vi "AB_1200_1100_Project_Source_ExportedAssemblyVI.vi"(7 "action":T4, 8 "error in (no error)":errorcluster, 9 "index in":i32, 10 "dataSource in":cluster{"ExportAssemblyVIinfo":T2}, 11 "buildObject":T1) -> (0 "error out":errorcluster, 1 "index out":i32, 2 "dataSource out":cluster{"ExportAssemblyVIinfo":T2}, 3 "buildObject out":T1)   [LabVIEW 2020]
doc: "Reads and writes the data to the object property bag."
uses:
  <vilib>/AppBuilder/RW_Project/AB_RW_Project_PropBag_Action.ctl
  <vilib>/AppBuilder/AB_InteropAssembly_DistVI_Proto_Info.ctl
  <vilib>/AppBuilder/IOStatus.ctl
  <resource>/Framework/Providers/API/ItemRef.ctl
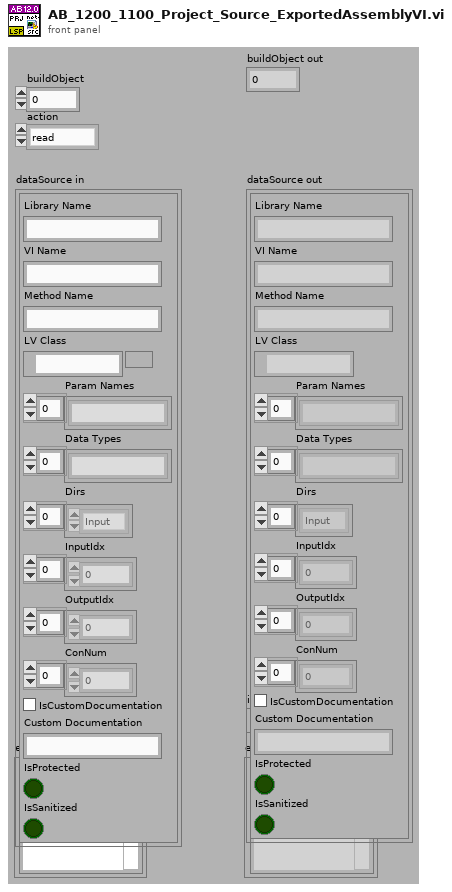
[diagram p1: front panel]
types:
  T1 = typedef "ItemRef.ctl" = u64
  T2 = typedef "AB_InteropAssembly_DistVI_Proto_Info.ctl" = cluster{"Library Name":string, "VI Name":string, "Method Name":string, "LV Class":path, "Param Names":string[], "Data Types":string[], "Dirs":T3[], "InputIdx":i32[], "OutputIdx":i32[], "ConNum":i8[], "IsCustomDocumentation":bool, "Custom Documentation":string, "IsProtected":bool, "IsSanitized":bool}
  T3 = typedef "IOStatus.ctl" = enum16{"Input", "Output", "Input/Output", "InputDeleted", "OutputDeleted", "IODeleted", "ErrorClusterIn", "ErrorClusterOut"}
  T4 = typedef "AB_RW_Project_PropBag_Action.ctl" = enum16{"read", "write", "clear", "readPrevious", "writePrevious", "clearPrevious"}
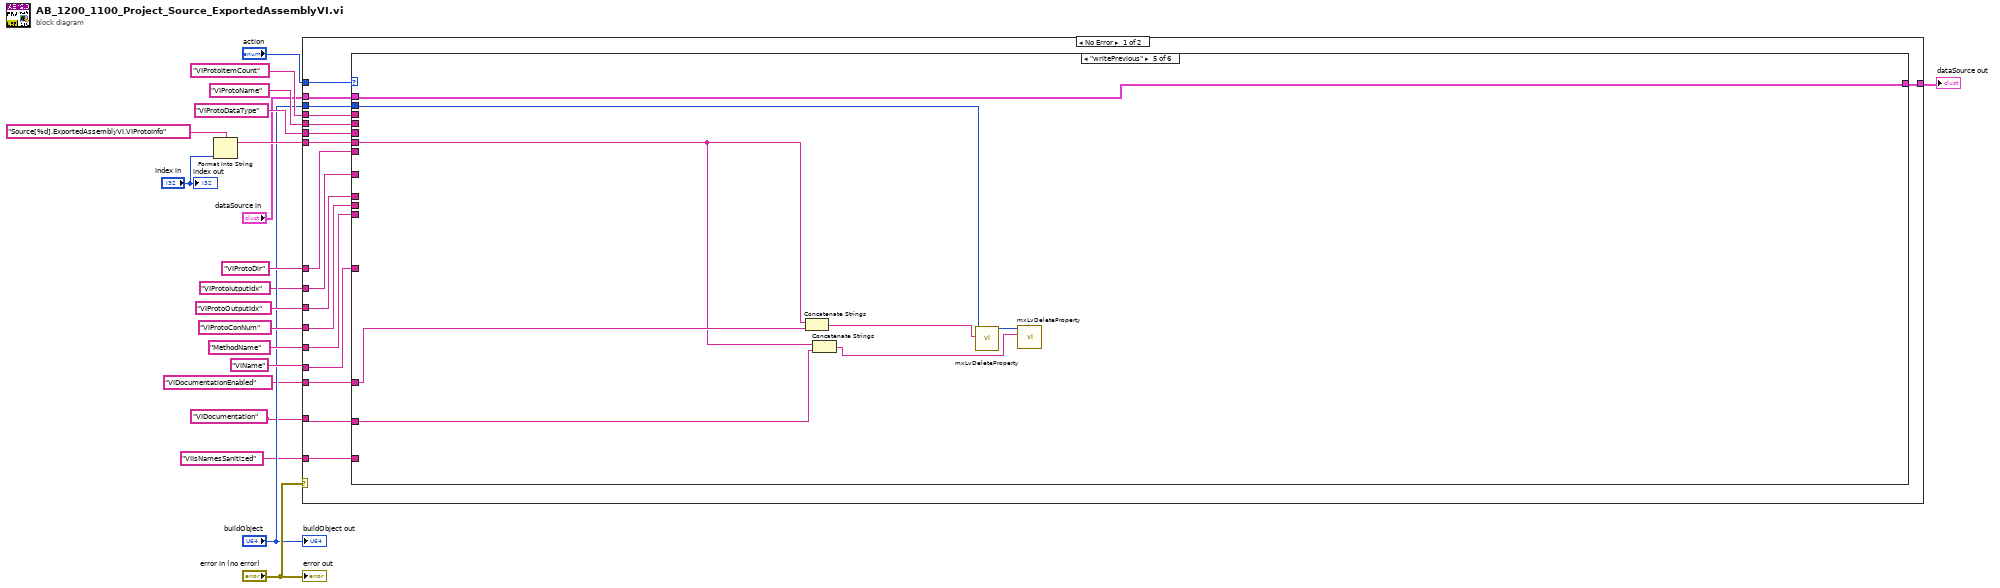
[diagram p0: block diagram]
diagram:
  n1 = Format Into String(format string="Source[%d].ExportedAssemblyVI.VIProtoInfo", "index in") -> (resulting string=w18:string)  [unwired: 2 in, 1 out]
  n2 = case shown="No Error" "error in (no error)" {
    tunnel: "action" -> [w37 _]
    tunnel: "dataSource in" -> [w36 w51]
    tunnel: w18 -> [w35 _]
    tunnel: "buildObject" -> [w34 _]
    tunnel: [w33 w51] -> w6
    tunnel: "VIProtoItemCount" -> [w32 _]
    tunnel: "VIProtoName" ("string") -> [w31 _]
    tunnel: "VIProtoDataType" ("string") -> [w30 _]
    tunnel: "VIProtoDir" ("string") -> [w29 _]
    tunnel: "VIProtoOutputIdx" ("string") -> [w28 _]
    tunnel: "VIProtoConNum" ("string") -> [w27 _]
    tunnel: "MethodName" -> [w26 _]
    tunnel: "VIName" -> [w25 _]
    tunnel: "VIProtoIutputIdx" ("string") -> [w24 _]
    tunnel: "VIDocumentation" -> [w23 _]
    tunnel: "VIDocumentationEnabled" -> [w22 _]
    tunnel: "VIIsNamesSanitized" -> [w21 _]
    frame No Error {
      n3 = case shown="\"writePrevious\"" w37 {
        tunnel: w34 -> [_ _ _ _ w45 _]
        tunnel: w36 -> [w38 w39 w40 w41 w49 w50]
        tunnel: w35 -> [_ _ _ _ w44 _]
        tunnel: [w38 w39 w40 w41 w49 w50] -> w33
        tunnel: w32 -> [_ _ _ _ _ _]
        tunnel: w31 -> [_ _ _ _ _ _]
        tunnel: w30 -> [_ _ _ _ _ _]
        tunnel: w29 -> [_ _ _ _ _ _]
        tunnel: w28 -> [_ _ _ _ _ _]
        tunnel: w27 -> [_ _ _ _ _ _]
        tunnel: w26 -> [_ _ _ _ _ _]
        tunnel: w25 -> [_ _ _ _ _ _]
        tunnel: w24 -> [_ _ _ _ _ _]
        tunnel: w23 -> [_ _ _ _ w43 _]
        tunnel: w22 -> [_ _ _ _ w48 _]
        tunnel: w21 -> [_ _ _ _ _ _]
        frame "read" {
        }
        frame "write" {
        }
        frame "clear" {
        }
        frame "readPrevious" {
        }
        frame "writePrevious" {
          n4 = Concatenate Strings(w44, w48) -> (w47:string)
          n5 = Concatenate Strings(w44, w43) -> (w42:string)
          n6 = call <resource>:"mxLvDeleteProperty.vi"("Tag"=w47, "Item"=w45) -> ("Item"=w46:T1)  [unwired: 2 in, 7 out]
          n7 = call <resource>:"mxLvDeleteProperty.vi"("Tag"=w42, "Item"=w46) -> ()  [unwired: 2 in, 8 out]
        }
        frame "clearPrevious" {
        }
      }
    }
    frame Error {
    }
  }
  "dataSource out" <- w6
  "error out" <- "error in (no error)"
  "index out" <- "index in"
  "buildObject out" <- "buildObject"
